vi "List Directory Recursive__ogtk.vi"(6 "List only Top-Level files in llbs? (FALSE)":bool, 8 "error in (no error)":errorcluster, 9 "Treat llb files as directories? (FALSE)":bool, 10 "pattern":string, 11 "Path":path) -> (0 "error out":errorcluster, 1 "dir paths":path[](array[path]), 2 "file paths":path[](array[path]), 3 "dup Path":path)   [LabVIEW 2012]
doc: "Returns an array of strings listing the names of all files in directory path and its subfolders, filtering the file names array based upon the specified pattern. If \"Treat llb files as directories\" is TRUE, llb files will not show up in the \"file paths\" output, but thier contents will. If \"List only Top-level files in llbs?\" is TRUE, only top-level llb contents will show up in the \"file paths\" output."
uses:
  <userlib>/_OpenG.lib/array/array.llb/Filter 1D Array (Path)__ogtk.vi
  <userlib>/_OpenG.lib/array/array.llb/Remove Duplicates from 1D Array (Path)__ogtk.vi
  <userlib>/_OpenG.lib/file/file.llb/Build Path - File Names Array__ogtk.vi
panel:
  # "[OpenG VI Tags] ***Do Not Remove***"
  # "List Recursive.vi\n\nGets an array of all files in dir and its sub-dir's\n\nPlease visit http://www.OpenG.org to learn about the\nOpen Source LabVIEW software movement.\n\nNOTICE -- YOU MUST LEAVE THIS NOTICE IN PLACE.  PER THE TERMS OF THE LICENSE BELOW, YOU MAY SUBLICENSE THIS SOFTWARE \nIN ANY WAY THAT DOES NOT CONFLICT WITH THIS LICENSE.\n\n### BSD License (http://www.opensource.org/licenses/bsd-license.php) Begin ###\n \nCopyright (c) 2002-2006, Jim Kring <jim@jimkring.com>\nCopyright (c) 2002, Cal-Bay Systems, Inc. <info@calbay.com>\n\nAll rights reserved.\n\nRedistribution and use in source and binary forms, with or without modification, are permitted provided that the following conditions are met:\n\n    * Redistributions of source code must retain the above copyright notice, this list of conditions and the following disclaimer.\n    * Redistributions in binary form must reproduce the above copyright notice, this list of conditions and the following disclaimer in the \n       documentation and/or other materials provided with the distribution.\n    * Neither the name of SciWare, James Kring, Inc., nor the names of its contributors may be used to endorse or promote products derived \n       from this software without specific prior written permission.\n\nTHIS SOFTWARE IS PROVIDED BY THE COPYRIGHT HOLDERS AND CONTRIBUTORS \"AS IS\" AND ANY EXPRESS OR IMPLIED WARRANTIES, \nINCLUDING, BUT NOT LIMITED TO, THE IMPLIED WARRANTIES OF MERCHANTABILITY AND FITNESS FOR A PARTICULAR PURPOSE ARE \nDISCLAIMED. IN NO EVENT SHALL THE COPYRIGHT OWNER OR CONTRIBUTORS BE LIABLE FOR ANY DIRECT, INDIRECT, INCIDENTAL,\n SPECIAL, EXEMPLARY, OR CONSEQUENTIAL DAMAGES (INCLUDING, BUT NOT LIMITED TO, PROCUREMENT OF SUBSTITUTE GOODS OR \nSERVICES; LOSS OF USE, DATA, OR PROFITS; OR BUSINESS INTERRUPTION) HOWEVER CAUSED AND ON ANY THEORY OF LIABILITY, \nWHETHER IN CONTRACT, STRICT LIABILITY, OR TORT (INCLUDING NEGLIGENCE OR OTHERWISE) ARISING IN ANY WAY OUT OF THE USE \nOF THIS SOFTWARE, EVEN IF ADVISED OF THE POSSIBILITY OF SUCH DAMAGE.\n\n### BSD License End ###"
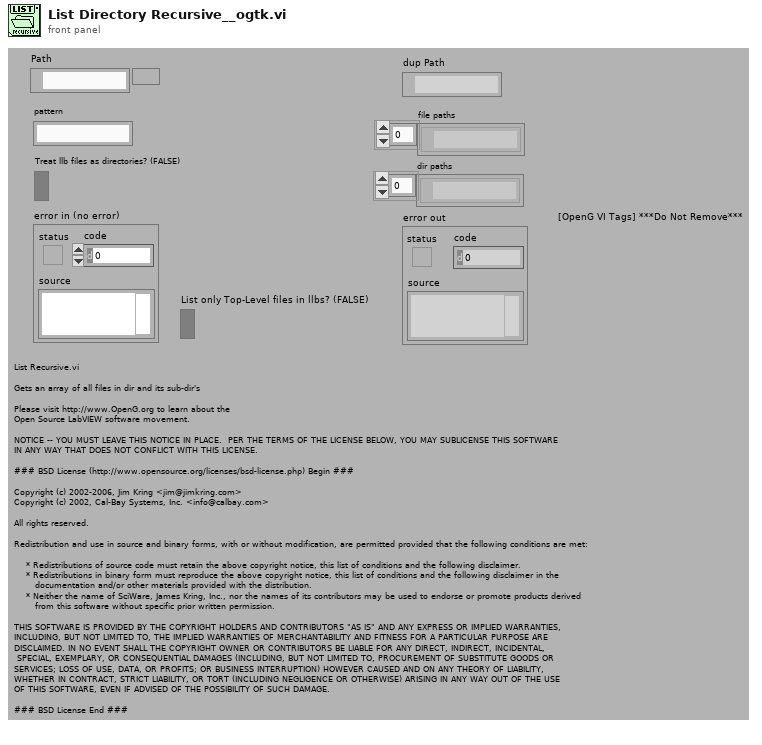
[diagram p1: front panel]
types:
  T1 = typedef "Librarian File Info Out.ctl" = cluster{"creation date":u32, "last mod date":u32, "type":string, "creator":string, "LV version":i32, "size":i32, "top level":bool}
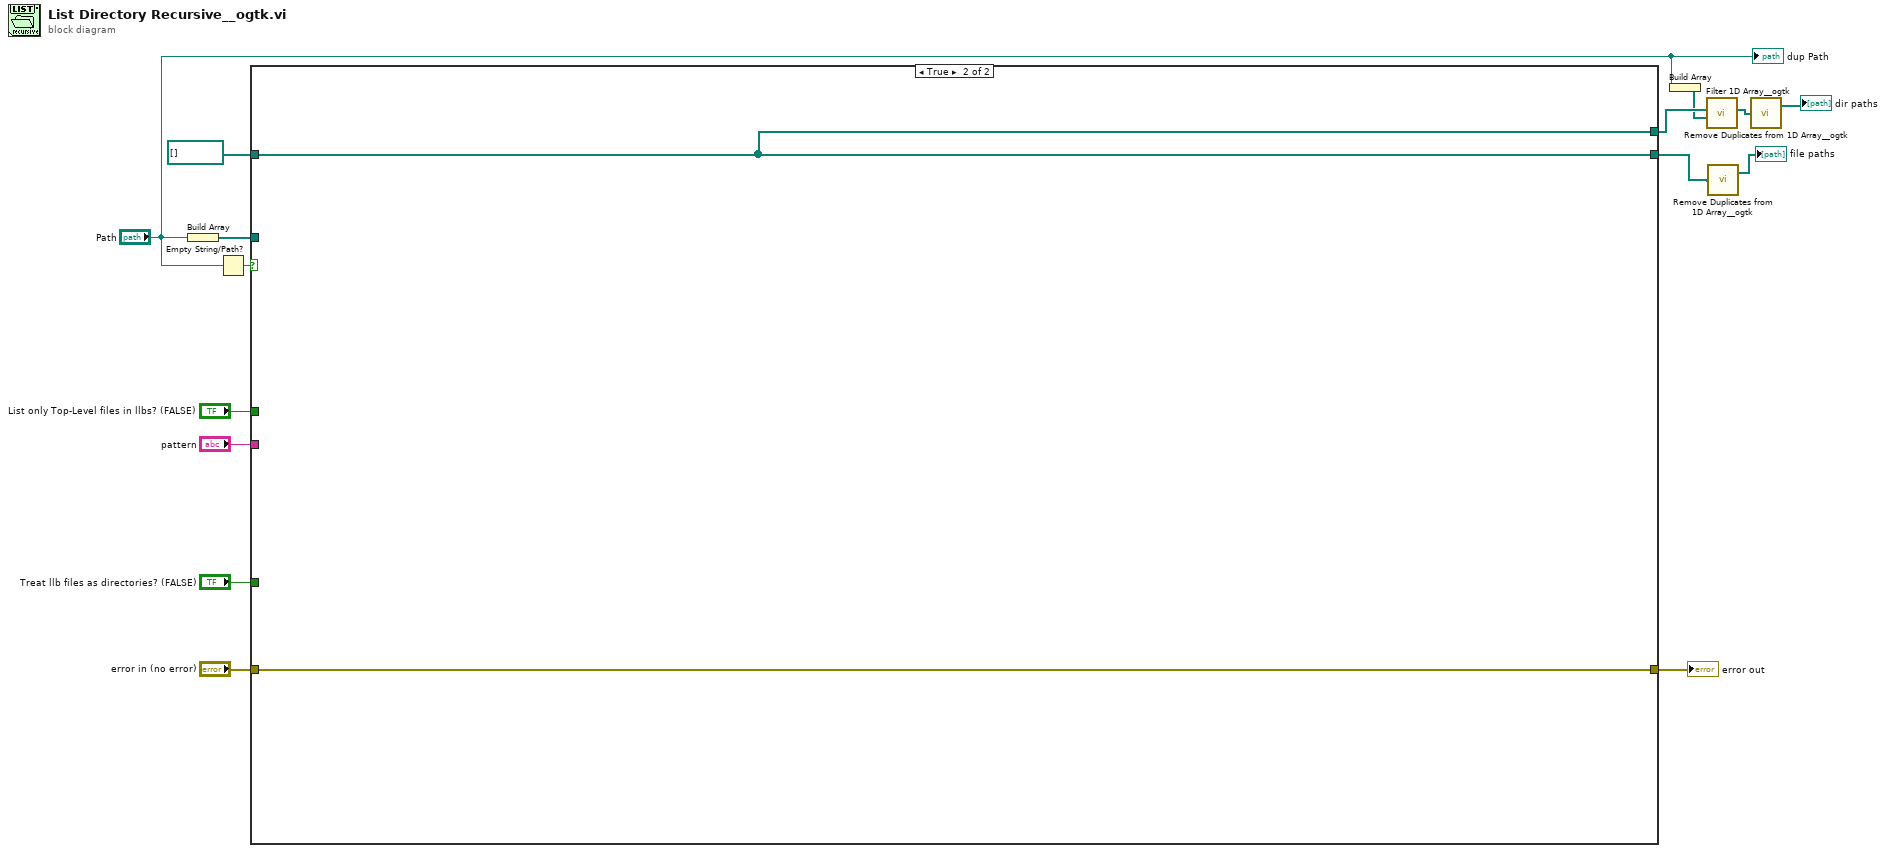
[diagram p0: block diagram]
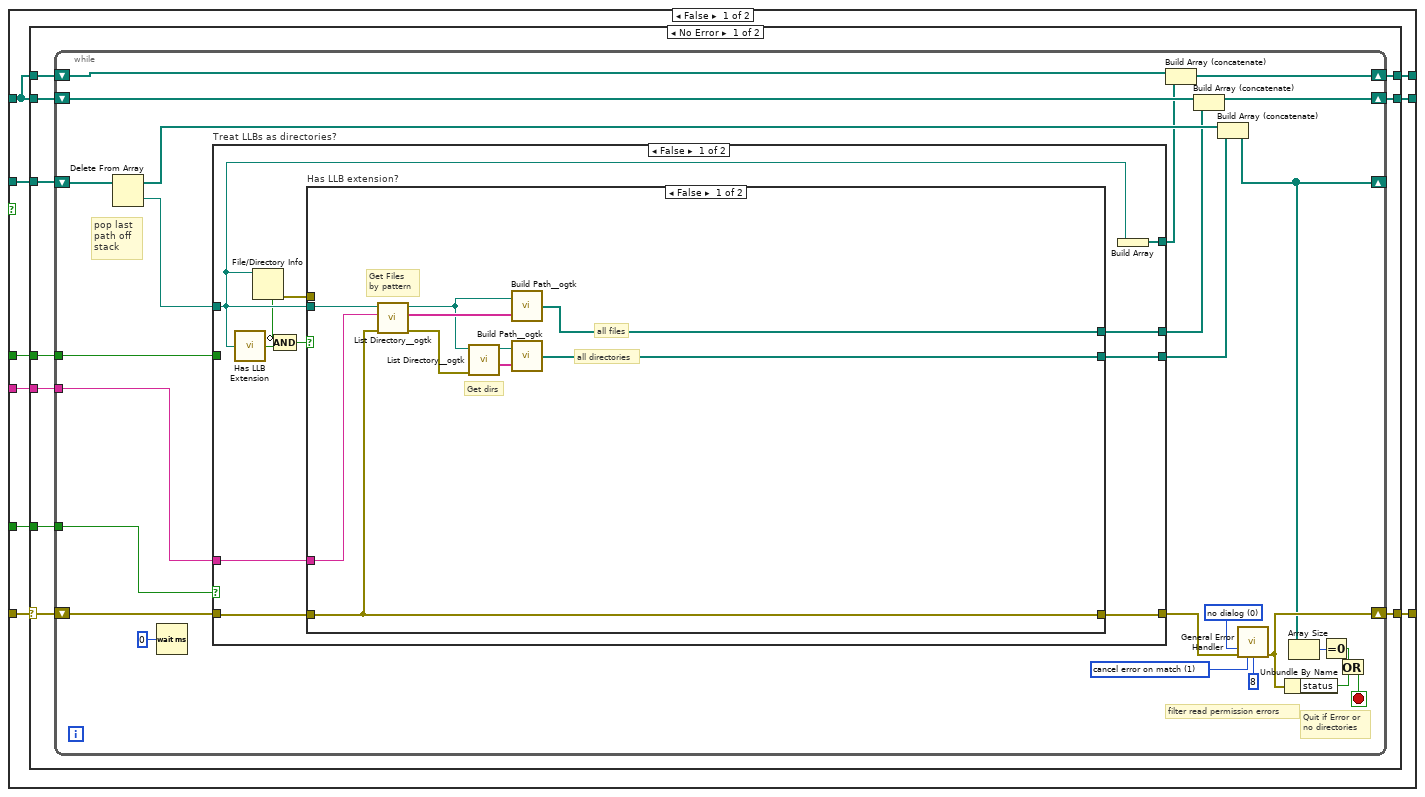
[diagram p2: hidden frame]
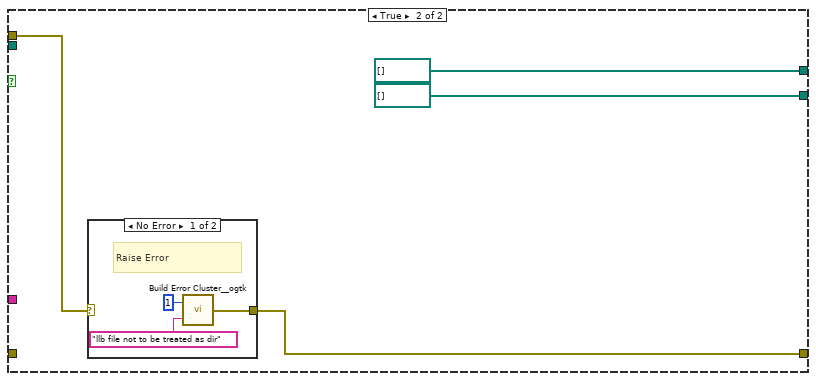
[diagram p3: hidden frame]
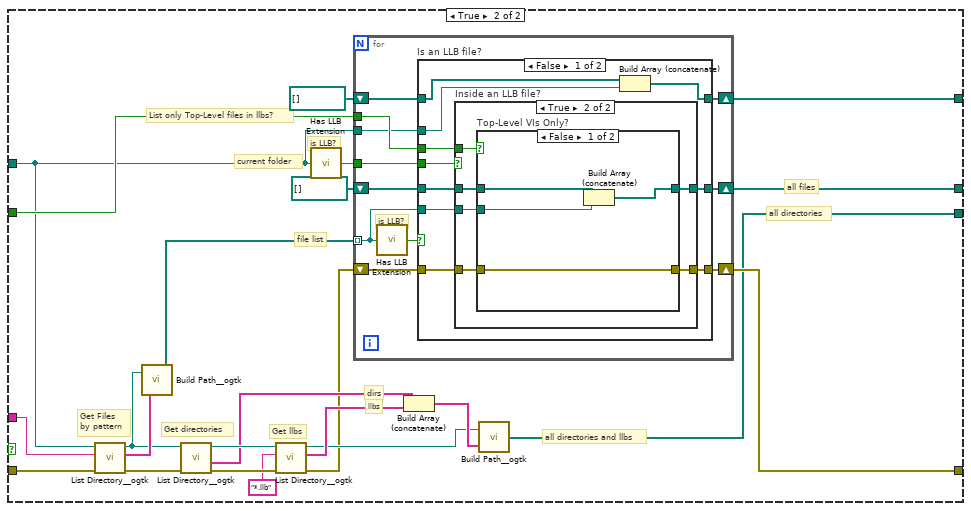
[diagram p5: hidden frame]
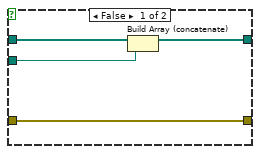
[diagram p6: hidden frame]
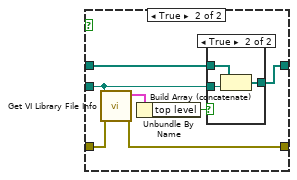
[diagram p7: hidden frame]
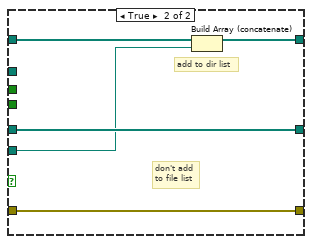
[diagram p9: hidden frame]
diagram:
  n1 = Build Array("Path") -> (w14:path[])
  n2 = Empty String/Path?(string/path="Path") -> (empty?=w8:bool)
  n3 = case shown="True" w8 {
    tunnel: [w24 w166] -> w15
    tunnel: w14 -> [w23 _]
    tunnel: path[] [] ("Array Constant") -> [w22 w167]
    tunnel: [w21 w167] -> w4
    tunnel: "pattern" -> [w20 _]
    tunnel: "Treat llb files as directories? (FALSE)" -> [w19 _]
    tunnel: "List only Top-Level files in llbs? (FALSE)" -> [w18 _]
    tunnel: "error in (no error)" -> [w17 w166]
    tunnel: [w16 w167] -> w7
    frame False {
      n4 = case shown="No Error" w17 {
        selector: w17 -> [w27 w165]
        tunnel: [w34 w165] -> w24
        tunnel: w23 -> [w33 _]
        tunnel: w22 -> [w32 w164]
        tunnel: [w31 w164] -> w21
        tunnel: w20 -> [w30 _]
        tunnel: w19 -> [w29 _]
        tunnel: w18 -> [w28 _]
        tunnel: w22 -> [w26 w163]
        tunnel: [w25 w163] -> w16
        frame No Error {
          n5 = while {
            shift-right: [w39] -> _
            shift-left: w33 -> [w54]
            shift-right: [w52] -> w34
            shift-left: w27 -> [w46]
            shift-right: [w49] -> w31
            shift-left: w32 -> [w53]
            tunnel: w30 -> [w45]
            tunnel: w29 -> [w40]
            tunnel: w28 -> [w41]
            shift-right: [w37] -> w25
            shift-left: w26 -> [w36]
            stop <- w55 stop-if-true
            w48 = u16 0 items=["no dialog", "OK message", "continue or stop message"] ("type of dialog (OK msg:1)")
            w51 = 1 items=["no exception", "cancel error on match", "set error on match"] ("[exception action] (none:0)")
            # "filter read permission errors"
            # "pop last path off stack"
            # "Quit if Error or no directories"
            n6 = Delete From Array(array=w54) -> (deleted portion=w59:path, array with subset deleted=w43:path[])  [unwired: 2 in]
            n7 = Wait (ms)(milliseconds to wait=u32 0) -> ()  [unwired: 1 out]
            n8 = case "Treat LLBs as directories?" shown="False" w40 {
              tunnel: w59 -> [w64 w90]
              tunnel: w46 -> [w70 w110]
              tunnel: [w69 w94] -> w38
              tunnel: w45 -> [w68 w111]
              tunnel: w41 -> [_ w96]
              tunnel: [w66 w93] -> w44
              tunnel: [w67 w92] -> w42
              tunnel: [w65 w89] -> w35
              frame False {
                n9 = call <vilib>:"Has LLB Extension.vi"("path"=w64) -> ("path to VI library?"=w63:bool)
                n10 = File/Directory Info(path=w64) -> (directory=w61:bool, error out=w60:errorcluster)  [unwired: 1 in, 5 out]
                n11 = Compound Arithmetic op=AND(invert w61, w63) -> (w62:bool)
                n12 = case "Has LLB extension?" shown="False" w62 {
                  tunnel: w70 -> [w77 _]
                  tunnel: [w77 w82] -> w69
                  tunnel: w64 -> [w78 _]
                  tunnel: w68 -> [w80 _]
                  tunnel: [w76 path[] [] ("appended path")] -> w67
                  tunnel: [w71 path[] [] ("appended path")] -> w66
                  tunnel: w60 -> [_ w81]
                  frame False {
                    # "Get dirs"
                    # "all directories"
                    # "all files"
                    # "Get Files\nby pattern"
                    n13 = call <userlib>:"List Directory__ogtk.vi"("error in (no error)"=w77, "pattern"=w80, "directory path"=w78) -> ("error out"=w75:errorcluster, "file names"=w79:string[], "dup directory path"=w74:path)  [unwired: 1 in, 1 out]
                    n14 = call <userlib>:"List Directory__ogtk.vi"("error in (no error)"=w75, "directory path"=w74) -> ("directory names"=w73:string[], "dup directory path"=w72:path)  [unwired: 2 in, 2 out]
                    n15 = call-poly <userlib>:"Build Path__ogtk.vi"("name or relative path"=w79, "base path"=w74) -> ("appended path"=w76:path[])
                    n16 = call-poly <userlib>:"Build Path__ogtk.vi"("name or relative path"=w73, "base path"=w72) -> ("appended path"=w71:path[])
                  }
                  frame True {
                    n17 = case shown="No Error" w81 {
                      selector: w81 -> [_ w88]
                      tunnel: [w85 w88] -> w82
                      frame No Error {
                        # "Raise Error"
                        n18 = call <userlib>:"Build Error Cluster__ogtk.vi"("String to Prepend to source (\"\")"="llb file not to be treated as dir" ("String to Prepend to source (\"\")"), "code"=1) -> ("error out"=w85:errorcluster)
                      }
                      frame Error {
                      }
                    }
                  }
                }
                n19 = Build Array(w64) -> (w65:path[])
              }
              frame True {
                # "all directories"
                # "all files"
                # "List only Top-Level files in llbs?"
                # "all directories and llbs"
                # "llbs"
                # "dirs"
                # "file list"
                # "is LLB?"
                # "current folder"
                # "Get llbs"
                # "Get directories"
                # "Get Files\nby pattern"
                n20 = call <userlib>:"List Directory__ogtk.vi"("error in (no error)"=w110, "pattern"=w111, "directory path"=w90) -> ("error out"=w99:errorcluster, "file names"=w109:string[], "dup directory path"=w98:path)  [unwired: 1 in, 1 out]
                n21 = call-poly <userlib>:"Build Path__ogtk.vi"("name or relative path"=w109, "base path"=w98) -> ("appended path"=w108:path[])
                n22 = call <userlib>:"List Directory__ogtk.vi"("error in (no error)"=w99, "directory path"=w98) -> ("error out"=w106:errorcluster, "directory names"=w102:string[], "dup directory path"=w103:path)  [unwired: 2 in, 1 out]
                n23 = call <userlib>:"List Directory__ogtk.vi"("error in (no error)"=w106, "pattern"="*.llb", "directory path"=w103) -> ("error out"=w95:errorcluster, "file names"=w104:string[], "dup directory path"=w100:path)  [unwired: 1 in, 1 out]
                n24 = call <vilib>:"Has LLB Extension.vi"("path"=w90) -> ("path to VI library?"=w97:bool)
                n25 = for {
                  tunnel: w108 -> [w121] mode=indexing
                  shift-right: [w120] -> w92
                  shift-left: path[] [] -> [w119]
                  tunnel: w97 -> [w118]
                  tunnel: w96 -> [w117]
                  shift-right: [w115] -> w94
                  shift-left: w95 -> [w116]
                  shift-right: [w113] -> w89
                  shift-left: path[] [] -> [w114]
                  tunnel: w90 -> [w112]
                  # "is LLB?"
                  n26 = call <vilib>:"Has LLB Extension.vi"("path"=w121) -> ("path to VI library?"=w122:bool)
                  n27 = case "Is an LLB file?" shown="False" w122 {
                    tunnel: w121 -> [w129 w159]
                    tunnel: [w128 w162] -> w120
                    tunnel: w119 -> [w130 w162]
                    tunnel: w118 -> [w132 _]
                    tunnel: w117 -> [w131 _]
                    tunnel: w116 -> [w127 w161]
                    tunnel: [w126 w161] -> w115
                    tunnel: w114 -> [w125 w160]
                    tunnel: [w124 w158] -> w113
                    tunnel: w112 -> [w123 _]
                    frame False {
                      n28 = case "Inside an LLB file?" shown="True" w132 {
                        tunnel: w131 -> [_ w142]
                        tunnel: w130 -> [w136 w141]
                        tunnel: w129 -> [w135 w140]
                        tunnel: [w134 w139] -> w128
                        tunnel: w127 -> [w133 w138]
                        tunnel: [w133 w137] -> w126
                        frame False {
                          n29 = Build Array (concatenate)(w136, w135) -> (w134:path[])
                        }
                        frame True {
                          n30 = case "Top-Level VIs Only?" shown="False" w142 {
                            tunnel: w140 -> [w145 w147]
                            tunnel: w141 -> [w146 w153]
                            tunnel: [w144 w152] -> w139
                            tunnel: w138 -> [w143 w150]
                            tunnel: [w143 w149] -> w137
                            frame False {
                              n31 = Build Array (concatenate)(w146, w145) -> (w144:path[])
                            }
                            frame True {
                              n32 = call <vilib>:"Get VI Library File Info.vi"("error in (no error)"=w150, "path"=w147) -> ("error out"=w149:errorcluster, "file information"=w148:T1)  [unwired: 8 in]
                              n33 = Unbundle By Name(w148) -> ("top level"=w151:bool)
                              n34 = case shown="True" w151 {
                                tunnel: w153 -> [w154 w157]
                                tunnel: w147 -> [_ w156]
                                tunnel: [w154 w155] -> w152
                                frame False {
                                }
                                frame True {
                                n35 = Build Array (concatenate)(w157, w156) -> (w155:path[])
                                }
                              }
                            }
                          }
                        }
                      }
                      n36 = Build Array (concatenate)(w125, w123) -> (w124:path[])
                    }
                    frame True {
                      # "add to dir list"
                      # "don't add\nto file list"
                      n37 = Build Array (concatenate)(w160, w159) -> (w158:path[])
                    }
                  }
                }
                n38 = Build Array (concatenate)(w102, w104) -> (w101:string[])
                n39 = call-poly <userlib>:"Build Path__ogtk.vi"("name or relative path"=w101, "base path"=w100) -> ("appended path"=w93:path[])
              }
            }
            n40 = Build Array (concatenate)(w36, w35) -> (w37:path[])
            n41 = Build Array (concatenate)(w53, w42) -> (w49:path[])
            n42 = Build Array (concatenate)(w43, w44) -> (w39:path[])
            n43 = call <vilib>:"General Error Handler.vi"("type of dialog (OK msg:1)"=w48, "error in (no error)"=w38, "[exception action] (none:0)"=w51, "[exception code]"=8) -> ("error out"=w52:errorcluster)  [unwired: 7 in, 4 out]
            n44 = Unbundle By Name(w52) -> ("status"=w57:bool)
            n45 = Array Size(array=w39) -> (size(s)=w58:i32)
            n46 = Equal To 0?(x=w58) -> (x = 0?=w56:bool)
            n47 = Or(x=w56, y=w57) -> (x .or. y?=w55:bool)
          }
        }
        frame Error {
        }
      }
    }
    frame True {
    }
  }
  "error out" <- w15
  n48 = Build Array("Path") -> (w5:path[])
  n49 = call-poly <userlib>:"Filter 1D Array__ogtk.vi"("items to filter"=w5, "array"=w7) -> ("filtered array"=w2:path[])  [unwired: 4 in, 1 out]
  n50 = call-poly <userlib>:"Remove Duplicates from 1D Array__ogtk.vi"("Input Array"=w4) -> ("Output Array"=→"file paths":path[])  [unwired: 1 out]
  n51 = call-poly <userlib>:"Remove Duplicates from 1D Array__ogtk.vi"("Input Array"=w2) -> ("Output Array"=→"dir paths":path[])  [unwired: 1 out]
  "dup Path" <- "Path"
